vi "Open Handle.vi"(0 "cookie file":path, 1 "BlueLogParent in":refnum<class "BlueLogParent_OpenSource.lvclass">, 5 "username":string, 7 "password":string, 11 "error IO":errorcluster, 12 "verify server(true)":bool=TRUE) -> (4 "client handle":T1, 15 "error IO":errorcluster)   [LabVIEW 2020, in "Blue Easy HTTP OpenSource.lvlib"]
uses:
  Blue Easy HTTP OpenSource.lvlib
  <vilib>/httpClient/ClientHandle.ctl
  <userlib>/Blue Origin/BlueLogParent_OpenSource/BlueLogParentClass/BlueLogParent_OpenSource.lvclass
  HTTP error on codes.ctl
  Interpret Header.vi
  <vilib>/dlg_ctls.llb/Space Constant.vi
  <vilib>/Utility/error.llb/Trim Whitespace.vi
  <vilib>/Utility/error.llb/Error Cluster From Error Code.vi
  <vilib>/httpClient/LabVIEWHTTPClient.lvlib
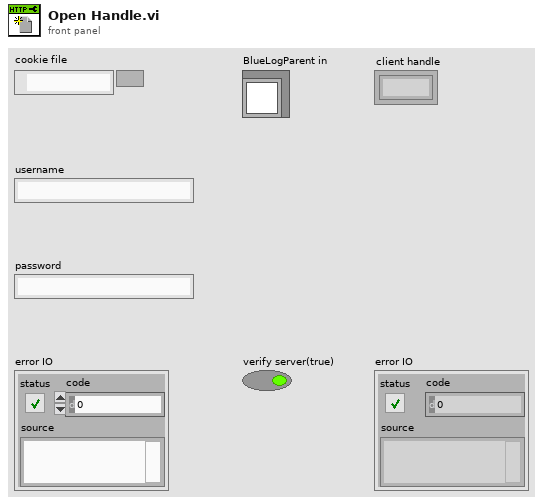
[diagram p1: front panel]
types:
  T1 = typedef "LabVIEWHTTPClient.lvlib/ClientHandle.ctl" = refnum<k1>
  T2 = typedef "Blue Easy HTTP OpenSource.lvlib/HTTP error on codes.ctl" = cluster{"1xx (info)":bool, "2xx (success)":bool, "3xx (redirect)":bool, "4xx (client error)":bool, "5xx (server error)":bool, "Other":bool}
  T3 = typedef "BlueLogParent_OpenSource.lvclass/BlueLogParentLevel.ctl" = enum16{"DEBUG", "INFO", "WARNING", "ERROR", "CRITICAL"}
  T4 = typedef "BlueLogParent_OpenSource.lvclass/BlueLogParentOptions.ctl" = cluster{"timestamp (now)":dbl, "Call chain (here)":string, "Count (1)":u16, "Font (override)":T5, "Add row separator? (T)":bool}
  T5 = typedef "BlueLogParent_OpenSource.lvclass/BlueLogParentFont.ctl" = cluster{"Font Name":string, "Size":u16, "Bold":bool, "Italic":bool, "Underline":bool, "Strikeout":bool, "Color":u32}
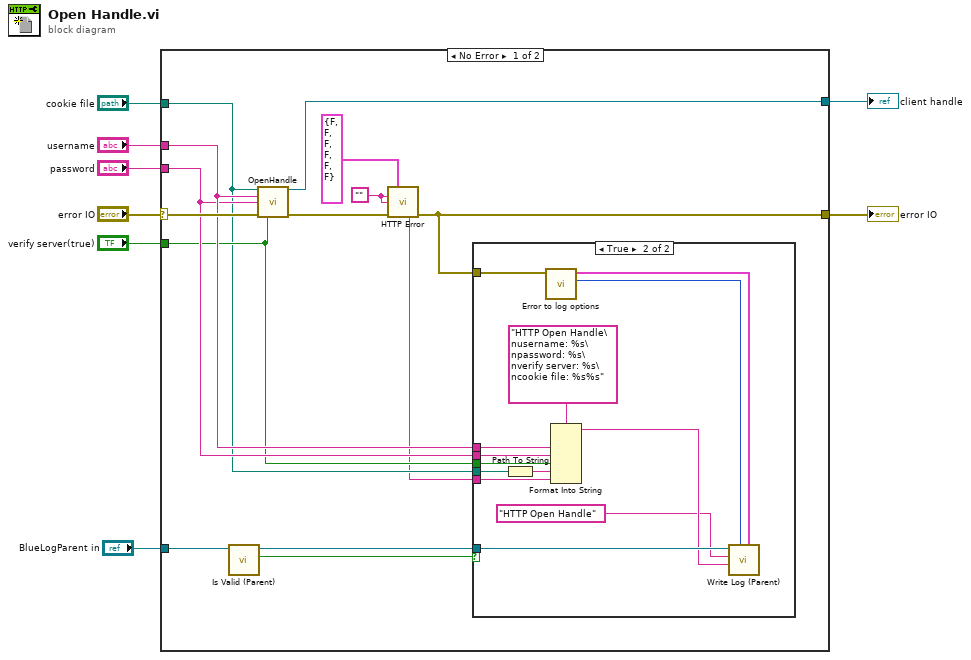
[diagram p0: block diagram]
diagram:
  n1 = case shown="No Error" "error IO" {
    selector: "error IO" -> [w22 w36]
    tunnel: [w9 w36] -> w7
    tunnel: [w21 _] -> w8
    tunnel: "cookie file" -> [w17 _]
    tunnel: "username" -> [w20 _]
    tunnel: "password" -> [w19 _]
    tunnel: "verify server(true)" -> [w18 _]
    tunnel: "BlueLogParent in" -> [w16 _]
    frame No Error {
      w10 = ""
      n2 = call-dynamic "Is Valid (Parent).vi"("BlueLogParent in"=w16) -> ("Is Valid?"=w15:bool, "BlueLogParent out"=w14:refnum<class "BlueLogParent_OpenSource.lvclass">)  [unwired: 8 in, 1 out]
      n3 = call <vilib>:"OpenHandle.vi"("cookie file"=w17, "username"=w20, "password"=w19, "error in (no error)"=w22, "verify server(true)"=w18) -> ("client handle out"=w21:T1, "error out"=w13:errorcluster)  [unwired: 9 in]
      n4 = call "HTTP Error.vi"("Error code options"=T2 {"1xx (info)"=FALSE, "2xx (success)"=FALSE, "3xx (redirect)"=FALSE, "4xx (client error)"=FALSE, "5xx (server error)"=FALSE, "Other"=FALSE}, "Header"=w10, "body"=w10, "error in (no error)"=w13) -> ("Error log"=w12:string, "error out"=w9:errorcluster)  [unwired: 6 in, 4 out]
      n5 = case shown="True" w15 {
        tunnel: w9 -> [_ w28]
        tunnel: w20 -> [_ w34]
        tunnel: w19 -> [_ w33]
        tunnel: w18 -> [_ w32]
        tunnel: w17 -> [_ w30]
        tunnel: w14 -> [_ w29]
        tunnel: w12 -> [_ w23]
        frame False {
        }
        frame True {
          n6 = Path To String(path=w30) -> (string=w31:string)
          n7 = call "Error to log options.vi"("error in (no error)"=w28) -> ("Logging level"=w26:T3, "Options"=w27:T4)  [unwired: 9 in]
          n8 = Format Into String(format string="HTTP Open Handle\nusername: %s\npassword: %s\nverify server: %s\ncookie file: %s%s", w34, w33, w32, w31, w23) -> (resulting string=w25:string)  [unwired: 2 in, 1 out]
          n9 = call-dynamic "Write Log (Parent).vi"("Options"=w27, "Logging level (INFO)"=w26, "Message"=w25, "Message Title"="HTTP Open Handle" ("Unique ID"), "BlueLogParent in"=w29) -> ()  [unwired: 5 in, 2 out]
        }
      }
    }
    frame Error {
    }
  }
  "client handle" <- w8
  "error IO" <- w7
